vi "SubPanel_Remove.vi"(8 "Error":errorcluster, 11 "SubPanel":refnum<vi>) -> (0 "Error Out":errorcluster, 3 "SubPanel Out":refnum<vi>)   [LabVIEW 2015]
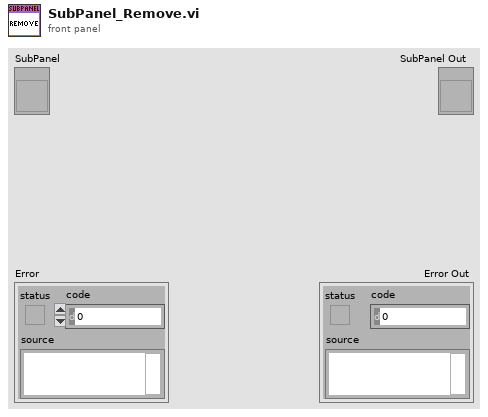
[diagram p1: front panel]
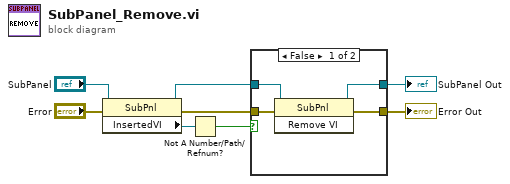
[diagram p0: block diagram]
diagram:
  n1 = property class="SubPnl"(reference="SubPanel", error in="Error") -> (reference out=w5:refnum<vi>, error out=w3:errorcluster, "InsertedVI"=w2:refnum<vi>)
  n2 = Not A Number/Path/Refnum?(number/path/refnum=w2) -> (NaN/Path/Refnum?=w1:bool)
  n3 = case shown="False" w1 {
    tunnel: [w12 w14] -> w8
    tunnel: [w11 w13] -> w7
    tunnel: w5 -> [w10 w13]
    tunnel: w3 -> [w9 w14]
    frame False {
      n4 = invoke class="SubPnl" method="Remove VI"(reference=w10, error in=w9) -> (reference out=w11:refnum<vi>, error out=w12:errorcluster)  [unwired: 1 in, 1 out]
    }
    frame True {
    }
  }
  "Error Out" <- w8
  "SubPanel Out" <- w7
